vi "Teleop.vi"(10 "Match Info":T1={"Autonomous Elapsed Seconds"=0.0, "TeleOp Elapsed Seconds"=0.0, "Disabled Elapsed Seconds"=0.0, "Visited Autonomous"=FALSE, "Visited TeleOp"=FALSE, "Visited Disabled"=FALSE, "Autonomous Settings"={"Autonomous Style"=enum."Independent", "VI Refnum"=refnum}}, 11 "Call Context":T2) -> ()   [LabVIEW 2014]
doc: "This VI is called for each TeleOp packet received from the DS where the robot is not disabled. It is often used to read from the joysticks and update I/O or to update setpoints for timed control loops. It should complete and return within 20 milliseconds or it may miss DS packets."
uses:
  <vilib>/Rock Robotics/WPI/DriverStation/WPI_DriverStationDerivedRobotMode.ctl
  <vilib>/Rock Robotics/WPI/DriverStation/WPI_DriverStationMatch Info.ctl
  Global Variables.vi
  <vilib>/Rock Robotics/WPI/Joystick/WPI_JoystickGetSetRefNum.vi
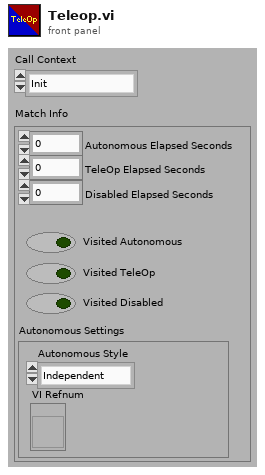
[diagram p1: front panel]
types:
  T1 = typedef "WPI_DriverStationMatch Info.ctl" = cluster{"Autonomous Elapsed Seconds":dbl, "TeleOp Elapsed Seconds":dbl, "Disabled Elapsed Seconds":dbl, "Visited Autonomous":bool, "Visited TeleOp":bool, "Visited Disabled":bool, "Autonomous Settings":cluster{"Autonomous Style":enum16{"Iterative", "Independent"}, "VI Refnum":refnum<vi>}}
  T2 = typedef "WPI_DriverStationDerivedRobotMode.ctl" = enum16{"Init", "Execute", "Stop"}
  T3 = typedef "WPI_JoystickDevRef.ctl" = cluster{"Device":T4}
  T4 = typedef "WPI_JoystickDeviceEnum.ctl" = enum16{"USB 0", "USB 1", "USB 2", "USB 3", "USB 4", "USB 5"}
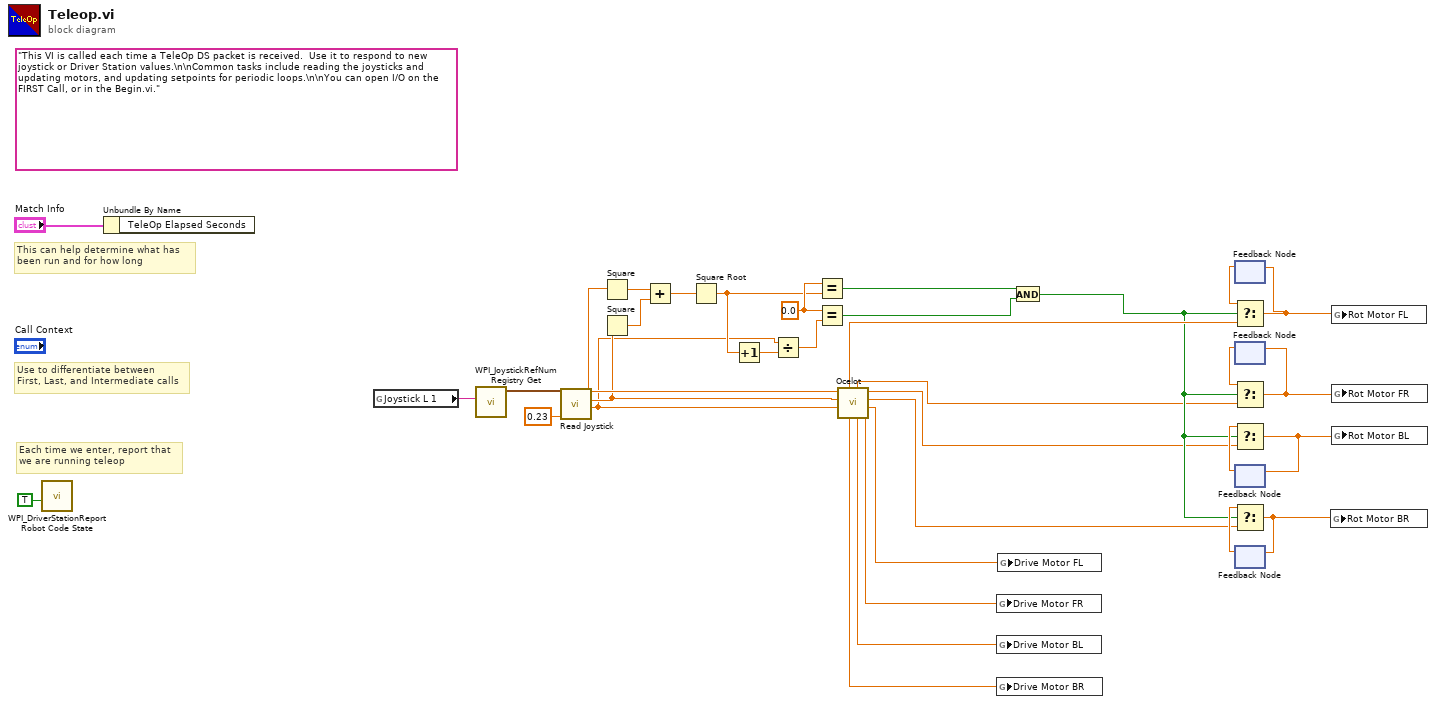
[diagram p0: block diagram]
diagram:
  w26 = 0.0 ("x")
  (unwired) "This VI is called each time a TeleOp DS packet is received.  Use it to respond to new joystick or Driver Station values.\n\nCommon tasks include reading the joysticks and updating motors, and updating setpoints for periodic loops.\n\nYou can open I/O on the FIRST Call, or in the Begin.vi."
  # "Each time we enter, report that\nwe are running teleop"
  # "Use to differentiate between\nFirst, Last, and Intermediate calls"
  # "This can help determine what has\nbeen run and for how long"
  n1 = call <vilib>:"WPI_DriverStationReport Robot Code State.vi"("TeleOp"=TRUE ("Autonomous")) -> ()  [unwired: 10 in, 1 out]
  n2 = Unbundle By Name("Match Info") -> ()  [unwired: 1 out]
  n3 = global read "Global Variables.vi" "Joystick L 1"() -> (w32:string)
  n4 = call <vilib>:"WPI_JoystickRefNum Registry Get.vi"("refnum name"=w32) -> ("JoystickDevRef"=w31:T3)  [unwired: 1 in, 9 out]
  n5 = call "Read Joystick.vi"("Joystick Deadbanded Value (default of 0.1)"=0.23, "Joystick L 1 DevRef"=w31) -> ("Joystick L 2 X Axis"=w1:dbl, "Joystick L 1 Y Axis"=w2:dbl, "Joystick L 1 X Axis"=w3:dbl)  [unwired: 7 in]
  n6 = Square(x=w3) -> (x^2=w28:dbl)
  n7 = Square(x=w2) -> (x^2=w29:dbl)
  n8 = Add(x=w28, y=w29) -> (x+y=w27:dbl)
  n9 = Square Root(x=w27) -> (sqrt(x)=w25:dbl)
  n10 = Increment(x=w25) -> (x+1=w24:dbl)
  n11 = Divide(x=w1, y=w24) -> (x/y=w23:dbl)
  n12 = Equal?(x=w26, y=w25) -> (x = y?=w17:bool)
  n13 = Equal?(x=w26, y=w23) -> (x = y?=w16:bool)
  n14 = call "Ocelot.vi"("RCW (X2)"=w1, "FWD (Y)"=w2, "STR (X)"=w3) -> ("FRD"=w6:dbl, "FLD"=w7:dbl, "BRS"=w8:dbl, "BLS"=w9:dbl, "BLD"=w5:dbl, "FRS"=w10:dbl, "BRD"=w4:dbl, "FLS"=w18:dbl)  [unwired: 1 in]
  n15 = global write "Global Variables.vi" "Drive Motor FR"(w6) -> ()
  n16 = global write "Global Variables.vi" "Drive Motor BL"(w5) -> ()
  n17 = global write "Global Variables.vi" "Drive Motor BR"(w4) -> ()
  n18 = global write "Global Variables.vi" "Drive Motor FL"(w7) -> ()
  n19 = And(x=w17, y=w16) -> (x .and. y?=w15:bool)
  n20 = feedback #1() -> (w22:dbl)  [unwired: 1 in]
  n21 = Select(t=w22, s=w15, f=w18) -> (s? t:f=w14:dbl)
  n22 = feedback-in #1(w14) -> ()
  n23 = feedback #2() -> (w21:dbl)  [unwired: 1 in]
  n24 = Select(t=w21, s=w15, f=w10) -> (s? t:f=w13:dbl)
  n25 = feedback-in #2(w13) -> ()
  n26 = feedback #3() -> (w20:dbl)  [unwired: 1 in]
  n27 = Select(t=w20, s=w15, f=w9) -> (s? t:f=w12:dbl)
  n28 = feedback-in #3(w12) -> ()
  n29 = feedback #4() -> (w19:dbl)  [unwired: 1 in]
  n30 = Select(t=w19, s=w15, f=w8) -> (s? t:f=w11:dbl)
  n31 = feedback-in #4(w11) -> ()
  n32 = global write "Global Variables.vi" "Rot Motor BR"(w11) -> ()
  n33 = global write "Global Variables.vi" "Rot Motor FL"(w14) -> ()
  n34 = global write "Global Variables.vi" "Rot Motor FR"(w13) -> ()
  n35 = global write "Global Variables.vi" "Rot Motor BL"(w12) -> ()
